vi "24HP_Create datalog header string.vi"() -> (0 "Datalog header string":string)   [LabVIEW 2020]
uses:
  <vilib>/Utility/error.llb/whitespace.ctl
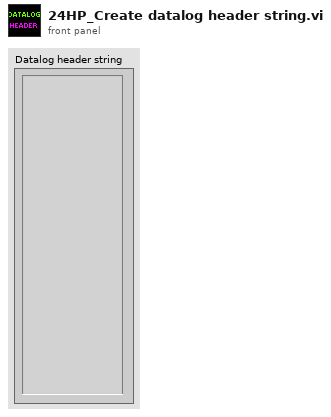
[diagram p1: front panel]
types:
  T1 = typedef "whitespace.ctl" = u16
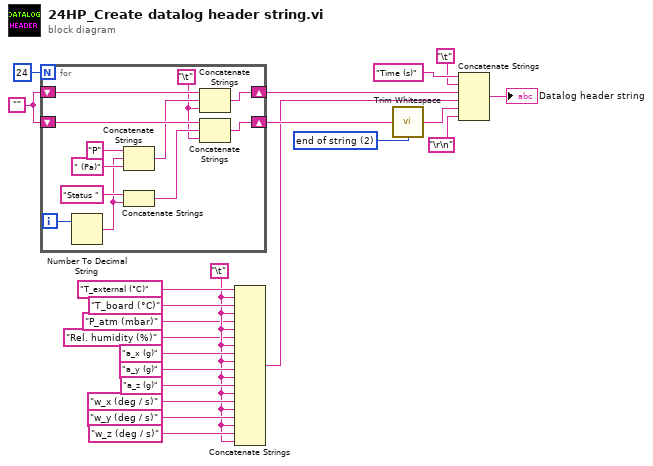
[diagram p0: block diagram]
diagram:
  w3 = "\t"
  w17 = T1 2 items=["both", "start of string", "end of string"] ("location (both)")
  w20 = ""
  n1 = for {
    N: 24 -> [_]
    shift-right: [w29] -> w16
    shift-left: w20 -> [w26]
    shift-right: [w28] -> w19
    shift-left: w20 -> [w27]
    i -> [w34]
    w23 = "\t"
    n2 = Number To Decimal String(number=w34) -> (decimal integer string=w30:string)  [unwired: 1 in]
    n3 = Concatenate Strings("P", w30, " (Pa)") -> (w25:string)
    n4 = Concatenate Strings("Status ", w30) -> (w24:string)
    n5 = Concatenate Strings(w27, w25, w23) -> (w28:string)
    n6 = Concatenate Strings(w26, w24, w23) -> (w29:string)
  }
  n7 = Concatenate Strings("T_external (°C)", w3, "T_board (°C)", w3, "P_atm (mbar)", w3, "Rel. humidity (%)", w3, "a_x (g)", w3, "a_y (g)", w3, "a_z (g)", w3, "w_x (deg / s)", w3, "w_y (deg / s)", w3, "w_z (deg / s)", w3) -> (w4:string)
  n8 = call <vilib>:"Trim Whitespace.vi"("string"=w16, "location (both)"=w17) -> ("trimmed string"=w15:string)
  n9 = Concatenate Strings("Time (s)", "\t", w19, w4, w15, "\r\n") -> (→"Datalog header string":string)
